vi "Sagar C V Half Adder and Full Adder.vi"() -> ()   [LabVIEW 2018]
panel:
  in  "?":string
  in  "?":string
  out "CARRY_FA":bool
  out "SUN_FA":bool
  out "CARRY_HA":bool
  out "SUN_HA":bool
  in  "Cin":bool
  in  "B":bool
  in  "A":bool
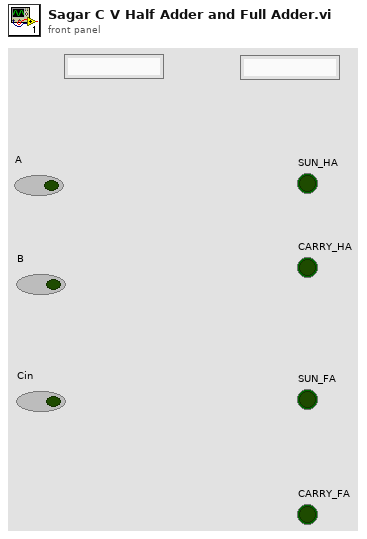
[diagram p1: front panel]
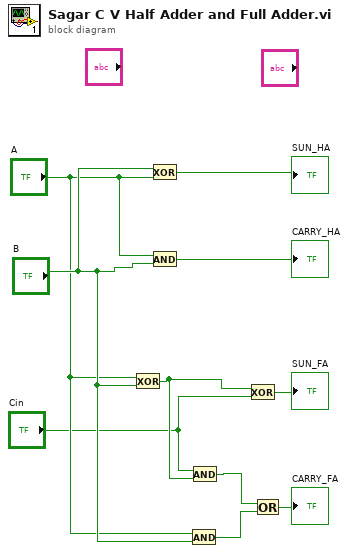
[diagram p0: block diagram]
diagram:
  n1 = Exclusive Or(1:"B", 2:"A") -> (0:w2:bool)
  n2 = Exclusive Or(1:"A", 2:"B") -> (0:→"SUN_HA":bool)
  n3 = And(x="A", y="B") -> (x .and. y?=→"CARRY_HA":bool)
  n4 = And(x="A", y="B") -> (x .and. y?=w5:bool)
  n5 = And(x="Cin", y=w2) -> (x .and. y?=w6:bool)
  n6 = Exclusive Or(1:"Cin", 2:w2) -> (0:→"SUN_FA":bool)
  n7 = Or(x=w6, y=w5) -> (x .or. y?=→"CARRY_FA":bool)
